vi "sub_resample_and_demodulate (User).vi"(4 "packet_array":cdb[][](array[numeric]), 5 "Rx IQ Sampling Rate [s/sec]":dbl, 6 "error in (no error)":errorcluster, 9 "PSK Init Parameters":T2) -> (0 "error out":errorcluster, 1 "recovered complex waveform":T1[](array[typedef]) {"Y" format="%.3f"; "dt" format="%^.2e"; "t0" format="%.4f"}, 2 "output bit stream":i8[][](array[numeric]), 3 "Sync Found":bool)   [LabVIEW 2013]
uses:
  <vilib>/addons/Modulation/Analog/controls/Complex Data Waveform.ctl
  <vilib>/addons/Modulation/niAMT.lvlib
  <vilib>/addons/Modulation/niDMT.lvlib
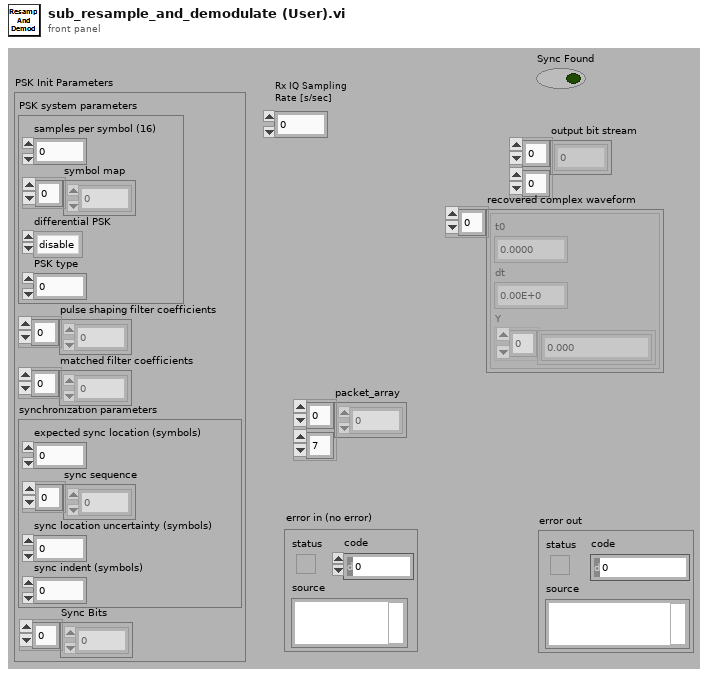
[diagram p1: front panel]
types:
  T1 = typedef "niAMT.lvlib/Complex Data Waveform.ctl" = cluster{"t0":dbl, "dt":dbl, "Y":cdb[]}
  T2 = cluster{"PSK system parameters":cluster{"samples per symbol (16)":i32, "symbol map":cdb[], "differential PSK":enum16{"disable", "enable"}, "PSK type":u16}, "pulse shaping filter coefficients":dbl[], "matched filter coefficients":dbl[], "synchronization parameters":cluster{"expected sync location (symbols)":i32, "sync sequence":cdb[], "sync location uncertainty (symbols)":i32, "sync indent (symbols)":i32}, "Sync Bits":i8[]}
  T3 = cluster{"samples per symbol (16)":i32, "symbol map":cdb[], "differential PSK":enum16{"disable", "enable"}, "PSK type":u16}
  T4 = cluster{"expected sync location (symbols)":i32, "sync sequence":cdb[], "sync location uncertainty (symbols)":i32, "sync indent (symbols)":i32}
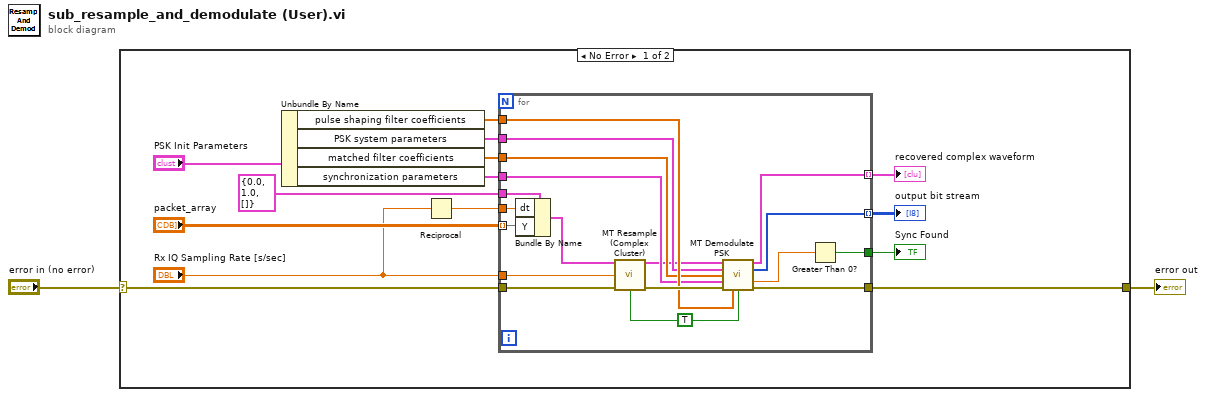
[diagram p0: block diagram]
diagram:
  n1 = case shown="No Error" "error in (no error)" {
    selector: "error in (no error)" -> [w6 w35]
    tunnel: [w5 w35] -> w2
    frame No Error {
      n2 = Unbundle By Name("PSK Init Parameters") -> ("pulse shaping filter coefficients"=w8:dbl[], "PSK system parameters"=w9:T3, "matched filter coefficients"=w10:dbl[], "synchronization parameters"=w11:T4)
      n3 = Reciprocal(x="Rx IQ Sampling Rate [s/sec]") -> (1/x=w3:dbl)
      n4 = for {
        tunnel: "packet_array" -> [w20] mode=indexing
        tunnel: "Rx IQ Sampling Rate [s/sec]" -> [w33]
        tunnel: w8 -> [w32]
        tunnel: w10 -> [w31]
        tunnel: w9 -> [w30]
        tunnel: [w29] -> w15 mode=indexing
        tunnel: w11 -> [w28]
        tunnel: [w26] -> w14
        tunnel: [w25] -> w5
        tunnel: [w17] -> w16 mode=indexing
        tunnel: w3 -> [w23]
        tunnel: T1 {"t0"=0.0, "dt"=1.0, "Y"=[]} ("input complex waveform") -> [w22]
        tunnel: w6 -> [w21]
        w24 = TRUE ("reset? (T)")
        n5 = Bundle By Name(cluster=w22, "dt"=w23, "Y"=w20) -> (w18:T1)
        n6 = call <vilib>:"MT Resample (Complex Cluster).vi"("input complex waveform"=w18, "desired sample rate (Hz)"=w33, "error in (no error)"=w21, "reset? (T)"=w24) -> ("output complex waveform"=w19:T1, "error out"=w34:errorcluster)  [unwired: 10 in]
        n7 = call <vilib>:"MT Demodulate PSK.vi"("input complex waveform"=w19, "PSK system parameters"=w30, "matched filter coefficients"=w31, "synchronization parameters"=w28, "error in (no error)"=w34, "pulse shaping filter coefficients"=w32, "reset? (T)"=w24) -> ("recovered complex waveform"=w17:T1, "output bit stream"=w29:i8[], "sync found index (symbols)"=w27:dbl, "error out"=w25:errorcluster)  [unwired: 4 in, 1 out]
        n8 = Greater Than 0?(x=w27) -> (x > 0?=w26:bool)
      }
      "Sync Found" <- w14
      "output bit stream" <- w15
      "recovered complex waveform" <- w16
    }
    frame Error {
    }
  }
  "error out" <- w2
